vi "closePistofono.vi"(8 "error in (no error)":errorcluster, 11 "Pistofono in":refnum<class "Pistofono.lvclass">) -> (0 "error out":errorcluster, 3 "Pistofono out":refnum<class "Pistofono.lvclass">)   [LabVIEW 2019, in "Pistofono.lvclass"]
uses:
  Pistofono.lvclass
  Pistofono.lvclass/Pistofono.ctl
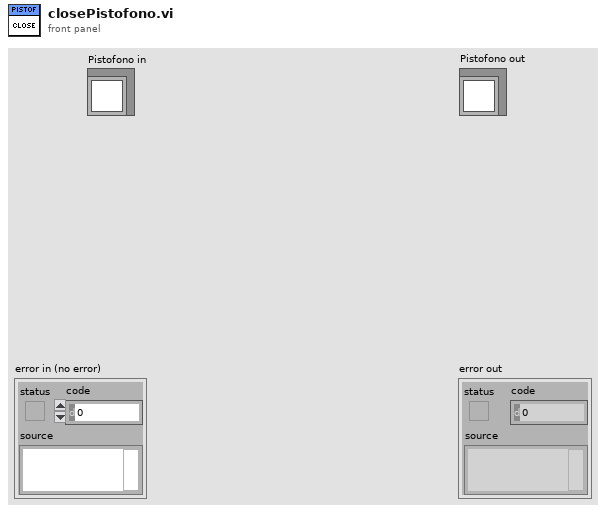
[diagram p1: front panel]
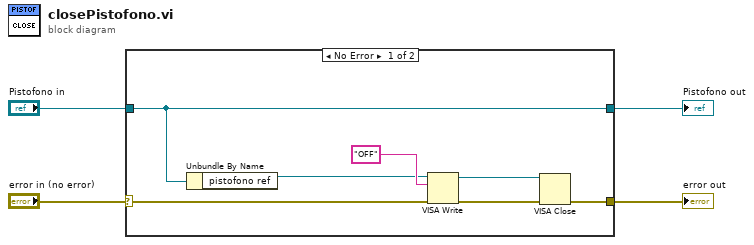
[diagram p0: block diagram]
diagram:
  n1 = case shown="No Error" "error in (no error)" {
    selector: "error in (no error)" -> [w5 w13]
    tunnel: [w11 w13] -> w3
    tunnel: [w10 w12] -> w1
    tunnel: "Pistofono in" -> [w10 w12]
    frame No Error {
      n2 = Unbundle By Name(w10) -> ("pistofono ref"=w8:refnum<visa-resource-name>)
      n3 = VISA Write(VISA resource name=w8, write buffer="OFF" ("Command"), error in (no error)=w5) -> (VISA resource name out=w7:refnum<visa-resource-name>, error out=w6:errorcluster)  [unwired: 1 out]
      n4 = VISA Close(VISA resource name=w7, error in (no error)=w6) -> (error out=w11:errorcluster)
    }
    frame Error {
    }
  }
  "error out" <- w3
  "Pistofono out" <- w1
